vi "Runtime True Constant.vi"(4 "Debug Value(F)":bool) -> (1 "Value":bool)   [LabVIEW 2017]
doc: "Returns a boolean constant. In the Run-Time Engine the output is always TRUE; in the development environment the constant is exposed so it can be changed while debugging."
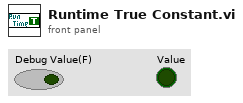
[diagram p1: front panel]
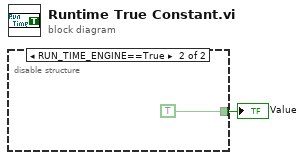
[diagram p0: block diagram]
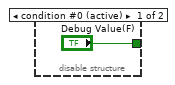
[diagram p2: hidden frame]
diagram:
  n1 = disable-structure shown="RUN_TIME_ENGINE==True" {
    disable-tunnel: ["Debug Value(F)" TRUE] -> w1
    frame condition #0 (active) {
    }
    frame condition #1 {
    }
  }
  "Value" <- w1
